vi "CLD 15 FGV for Text String Parsing Exercise.vi"(8 "Fehler (Eingang)":T2, 11 "Modus":T3) -> (0 "Fehler (Ausgang)":T2)   [LabVIEW 2009]
doc: "CLD 15 - Mit diesem VI werden die Datei ausgelesen. Die Daten der Datei werden mit Hilfe von zwei Sub-VIs für die weitere Verwendung analysiert und anschließend formatiert."
uses:
  CLD 15 CSV file data structure.ctl
  CLD 15 CSV file enum.ctl
panel:
  out "Formatierte Daten (Ausgang)":T1[](array[typedef])
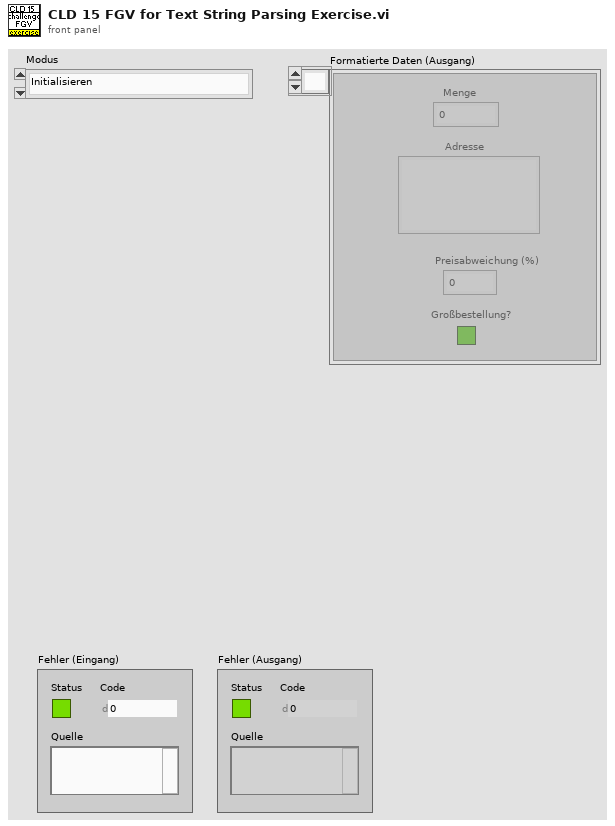
[diagram p1: front panel]
types:
  T1 = typedef "CLD 15 CSV file data structure.ctl" = cluster{"Menge":i32, "Adresse":string, "Preisabweichung (%)":dbl, "Großbestellung?":bool}
  T2 = cluster{"Status":bool, "Code":i32, "Quelle":string}
  T3 = typedef "CLD 15 CSV file enum.ctl" = enum16{"Initialisieren", "CSV lesen", "Daten verarbeiten", "CSV schreiben"}
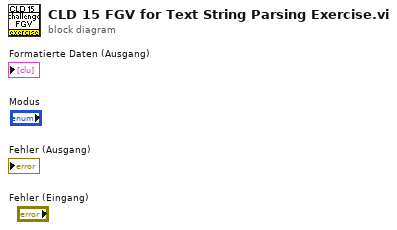
[diagram p0: block diagram]
diagram:
